vi "Cache_Info Global_Load All.vi"(8 "error in (no error)":errorcluster) -> (0 "error out":errorcluster, 1 "All Success?":bool, 2 "Interface Info":map{string, bool}(c390), 3 "Info":map{string, T1}(c390))   [LabVIEW 2019, in "ClassLoader.lvlib"]
uses:
  ClassLoader.lvlib
  <vilib>/Utility/config.llb/NI_LVConfig.lvlib
  Cache_Info Global.vi
  Ctl/Ctl_Class Info.ctl
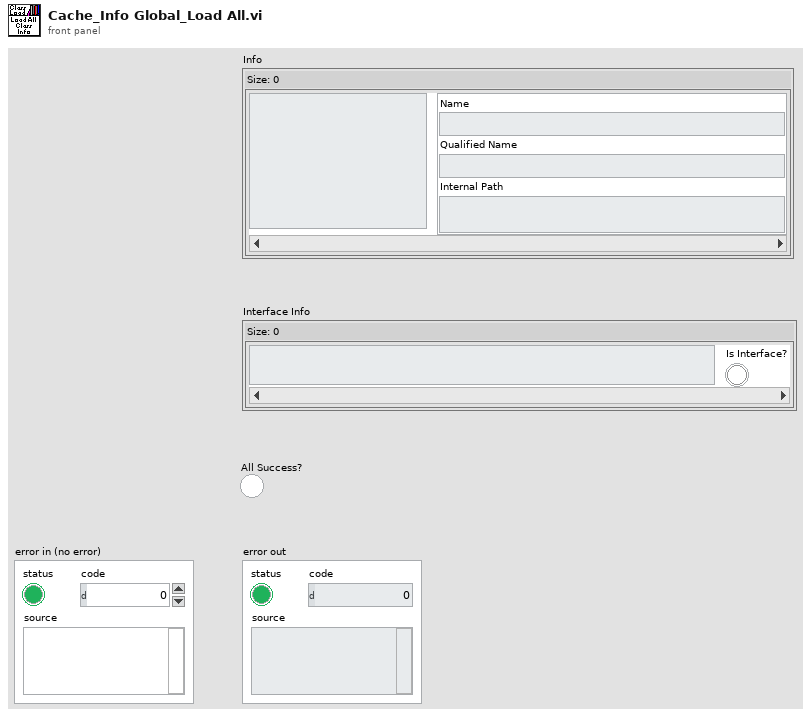
[diagram p1: front panel]
types:
  T1 = typedef "ClassLoader.lvlib/Ctl_Class Info.ctl" = cluster{"Name":string, "Qualified Name":string, "Internal Path":string}
  T2 = typedef "NI_LVConfig.lvlib/Config Data RefNum.ctl" = refnum<k1>
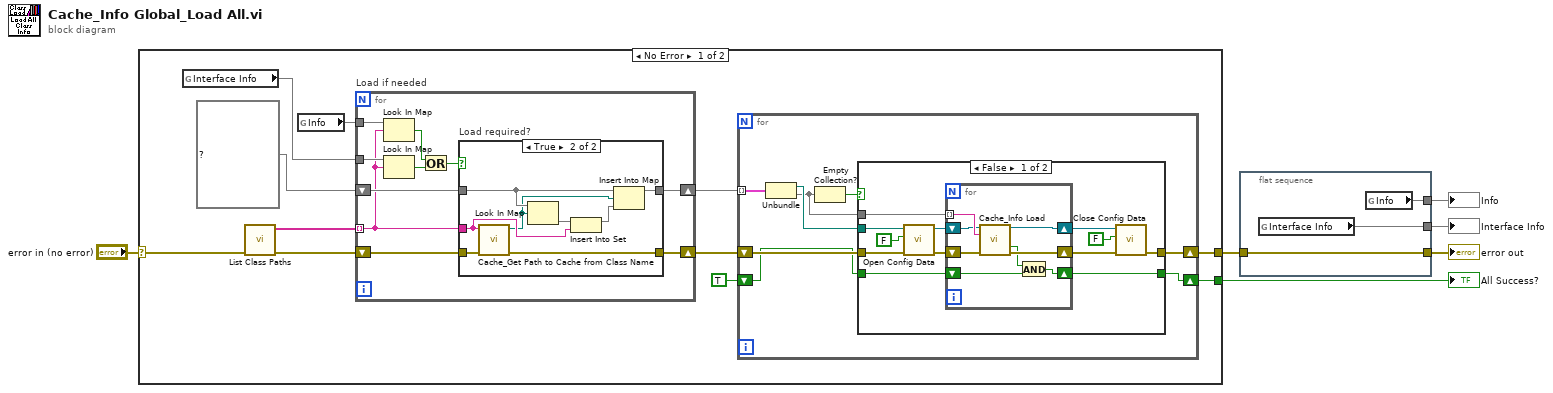
[diagram p0: block diagram]
diagram:
  n1 = case shown="No Error" "error in (no error)" {
    selector: "error in (no error)" -> [w17 w68]
    tunnel: [w11 w68] -> w4
    tunnel: [w9 _] -> w3
    frame No Error {
      n2 = global read "Cache_Info Global.vi" "Interface Info"() -> (w7:map{string, bool})
      n3 = call "List Class Paths.vi"("error in (no error)"=w17) -> ("error out"=w13:errorcluster, "Class Names"=w16:string[])  [unwired: 8 in, 1 out]
      n4 = global read "Cache_Info Global.vi" "Info"() -> (w8:map{string, T1})
      n5 = for "Load if needed" {
        tunnel: w16 -> [w48] mode=indexing
        tunnel: w8 -> [w56]
        shift-right: [w54] -> w12
        shift-left: map{path, set{string}} {} ("map") -> [w55]
        shift-right: [w53] -> w14
        shift-left: w13 -> [w52]
        tunnel: w7 -> [w51]
        n6 = Look In Map(map=w56, key=w48) -> (key not found?=w57:bool)  [unwired: 1 in, 1 out]
        n7 = Look In Map(map=w51, key=w48) -> (key not found?=w49:bool)  [unwired: 1 in, 1 out]
        n8 = Or(x=w57, y=w49) -> (x .or. y?=w50:bool)
        n9 = case "Load required?" shown="True" w50 {
          tunnel: w48 -> [_ w66]
          tunnel: w55 -> [w59 w65]
          tunnel: [w59 w64] -> w54
          tunnel: [w58 w60] -> w53
          tunnel: w52 -> [w58 w61]
          frame False {
          }
          frame True {
            n10 = call "Cache_Get Path to Cache from Class Name.vi"("error in (no error)"=w61, "Class Name"=w66) -> ("error out"=w60:errorcluster, "Cache Path"=w63:path)  [unwired: 7 in, 1 out]
            n11 = Look In Map(map=w65, key=w63) -> (value=w67:set{string})  [unwired: 1 in, 1 out]
            n12 = Insert Into Set(10:w66, 11:w67) -> (3:w62:set{string})  [unwired: 1 out]
            n13 = Insert Into Map(map in=w65, key=w63, value=w62) -> (map out=w64:map{path, set{string}})  [unwired: 2 out]
          }
        }
      }
      n14 = for {
        tunnel: w12 -> [w25] mode=indexing
        shift-right: [w22] -> w11
        shift-left: w14 -> [w23]
        shift-right: [w18] -> w9
        shift-left: TRUE -> [w19]
        n15 = Unbundle(w25) -> ("Cache Path"=w24:path, "set"=w21:set{string})
        n16 = Empty Collection?(1:w21) -> (0:w20:bool)
        n17 = case shown="False" w20 {
          tunnel: w24 -> [w36 _]
          tunnel: w23 -> [w35 w47]
          tunnel: [w29 w47] -> w22
          tunnel: w21 -> [w28 _]
          tunnel: w19 -> [w27 w46]
          tunnel: [w26 w46] -> w18
          frame False {
            n18 = call <vilib>:"Open Config Data.vi"("error in (no error)"=w35, "create file if necessary (T)"=FALSE, "configuration file path"=w36) -> ("error out"=w31:errorcluster, "refnum"=w33:T2)  [unwired: 6 in, 1 out]
            n19 = for {
              shift-right: [w43] -> w32
              shift-left: w33 -> [w44]
              tunnel: w28 -> [w45] mode=indexing
              shift-right: [w41] -> w30
              shift-left: w31 -> [w42]
              shift-right: [w38] -> w26
              shift-left: w27 -> [w40]
              n20 = call "Cache_Info Load.vi"("Refnum in"=w44, "Class Name"=w45, "error in (no error)"=w42) -> ("Refnum out"=w43:T2, "Success?"=w39:bool, "error out"=w41:errorcluster)  [unwired: 8 in, 2 out]
              n21 = And(x=w39, y=w40) -> (x .and. y?=w38:bool)
            }
            n22 = call <vilib>:"Close Config Data.vi"("error in (no error)"=w30, "write file if changed (T)"=FALSE, "refnum"=w32) -> ("error out"=w29:errorcluster)  [unwired: 7 in, 1 out]
          }
          frame True {
          }
        }
      }
    }
    frame Error {
    }
  }
  "All Success?" <- w3
  n23 = flat-sequence {
    tunnel: [w71] -> w5
    tunnel: w4 -> [w71]
    tunnel: [w70] -> w2
    tunnel: [w69] -> w1
    frame #0 {
      n24 = global read "Cache_Info Global.vi" "Interface Info"() -> (w69:map{string, bool})
      n25 = global read "Cache_Info Global.vi" "Info"() -> (w70:map{string, T1})
    }
  }
  "error out" <- w5
  "Info" <- w2
  "Interface Info" <- w1
